vi "Trajectory Builder.vi"() -> ()   [LabVIEW 2020]
uses:
  Availible Command systems for auto.ctl
  <vilib>/event_ctls.llb/lveventtype.ctl
panel:
  out "Picture":picture
  in  "Initial Location":cluster{"x":dbl, "y":dbl, "th":dbl}[](array[cluster])=[{"x"=9.6, "y"=6.2, "th"=90.0}]
  out "appended path":path
  out "folder names":cluster{"name":string, "name":string}
  in  "Directory":bool
  in  "Tab Control":T1(tab)
  out "Duration (s)":dbl format="%#.4g"
  out "Distance (ft)":dbl format="%#.1g"
  out "WayPoints":cluster{"x":dbl, "y":dbl, "th":dbl}[](array[cluster]) {"th" format="%#_4g"}
  in  "Center Flip":bool
  in  "Snap to foot":bool
  in  "Angle Limiter":enum16{"90", "45", "15", "1"}(ring)=enum."15"
  in  "Snap robot to baseline":bool
  in  "Angular Accelerations":T2 {"Angular \nAccelerations" step=5.0}
  in  "Limits":T3={"Velocity (fps)"=6.0, "Accel (fps^2)"=15.0, "Jerk (fps^3)"=15.0} {"Jerk (fps^3)" min=0.0 step=1.0; "Accel (fps^2)" min=0.0; "Velocity (fps)" min=0.0}
  in  "Conditions":T4 {"vFinal (fps)" min=0.0; "vInitial (fps)" min=0.0}
  in  "Sample Period (s)":dbl=0.02
  in  "Unjank":bool
  in  "Turn \nAcceleration":bool=TRUE
  in  "Turn \nDeceleration":bool=TRUE
  out "Command Info":string
  in  "Reorder":bool
  in  "Commands":T5(array[cluster]) {"System" items=["Elevator", "Carriage Intake STOP", "Carriage Intake RUN"]}
  in  "Time (s)":dbl(slide) scale=-1.0..2.02 scale format="%#.1g"
  in  "Play":bool
  in  "Sub Dir 2":u16(ring)
  in  "Sub Dir 1":u16(ring) items=["Experimental", "Left", "Other", "Right"]
  out "fps":dbl[](graph)
  in  "Append":bool
  in  "Open":i32(listbox)
  in  "Filename":string
  in  "Save":bool
  in  "New":bool
  # "Directions:\nUse mouse to ...\n    move robot position (rectangle with arrow)\n    rotate robot (red arrow)\n    move waypoints (numbered circles)\nClick in open space to add a waypoint\nShift click to delete a waypoint\nHover over a waypoint and use arrow keys to nudge\n\nTime slider and Play button will run robot along path\nto test for collisions\n\nDirection and Destionation are folder selectors for files\n\nNew creates a new path at default location\n\nAppend creates a path"
  # "Nicotine"
  # "(20ms)"
  # "Interaction Options"
  # "Path Info"
  # "1"
  # "2"
  # "3"
  # "4"
  # "5"
  # "6"
  # "7"
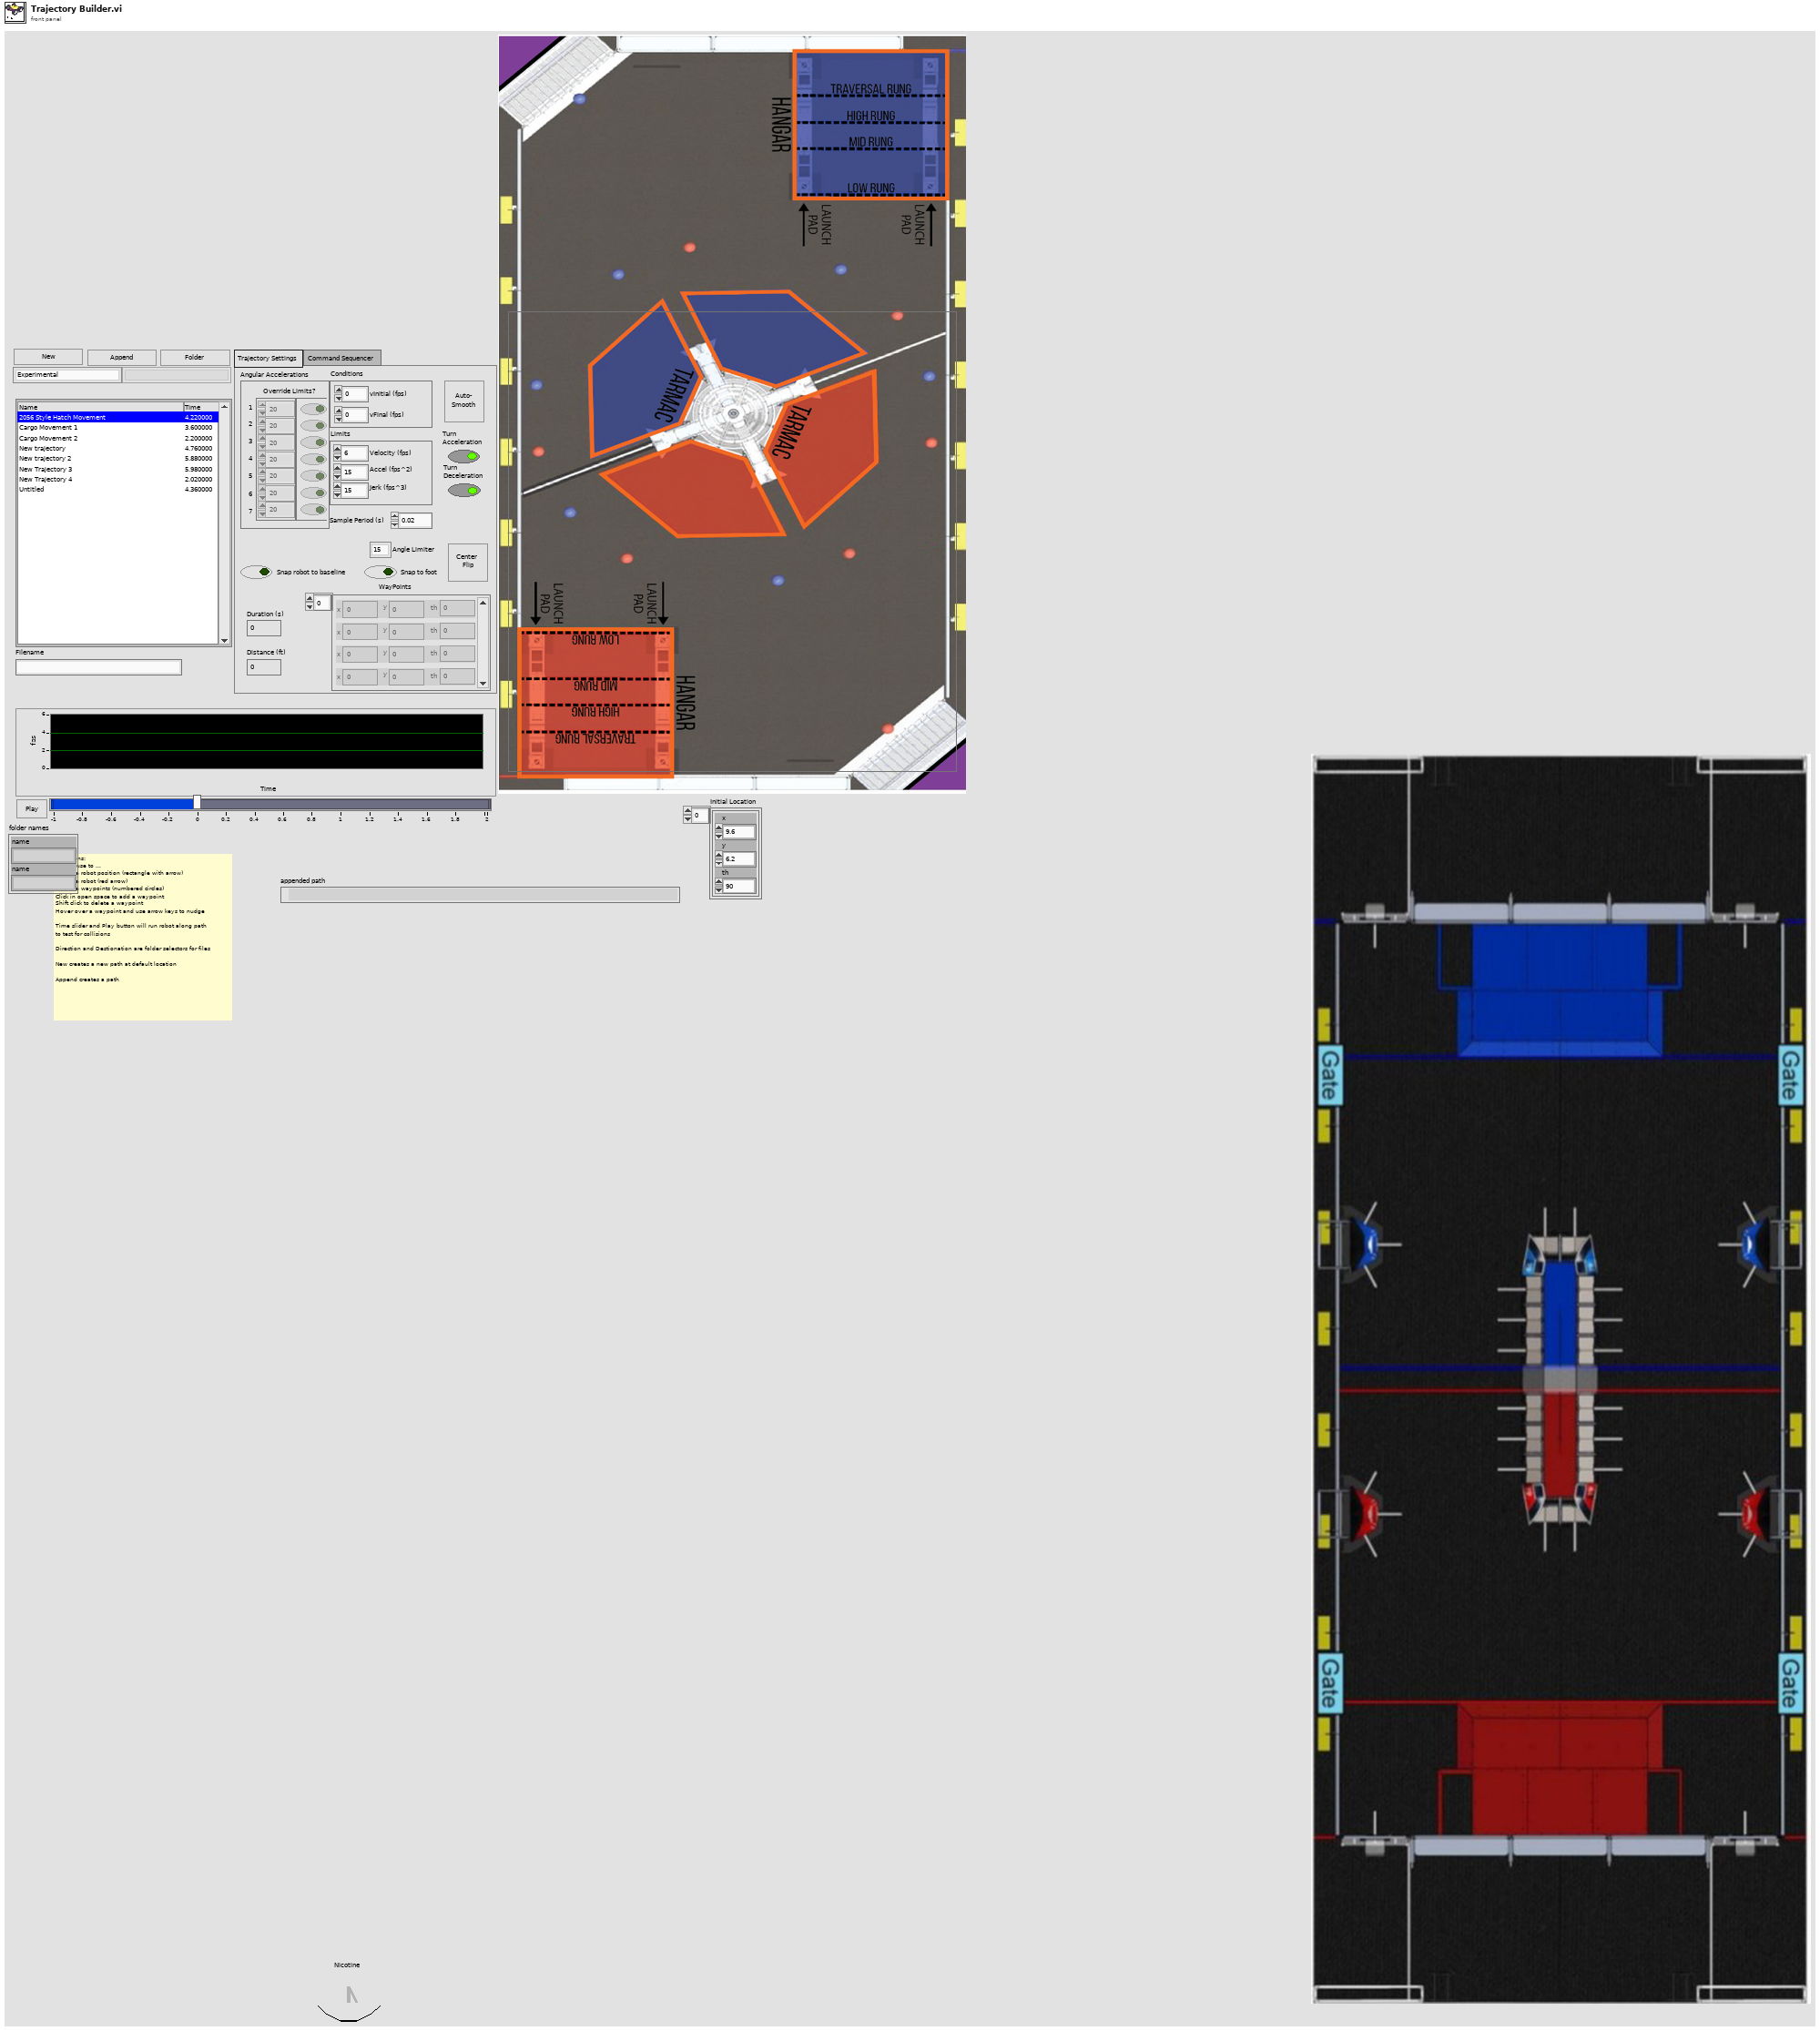
[diagram p1: front panel]
types:
  T1 = enum32{"Trajectory Settings", "Command Sequencer"}
  T2 = cluster{"Angular \nAccelerations":dbl[], "Override Limits?":bool[]}
  T3 = cluster{"Velocity (fps)":dbl, "Accel (fps^2)":dbl, "Jerk (fps^3)":dbl}
  T4 = cluster{"vInitial (fps)":dbl, "vFinal (fps)":dbl}
  T5 = cluster{"Time into Path":dbl, "System":u16, "Item Selected?":bool, "System Selection":u16}[]
  T6 = cluster{"Sample Period (s)":dbl, "Limits":cluster{"Velocity (fps)":dbl, "Acceleration (fps^2)":dbl, "Jerk (fps^3)":dbl}, "Conditions":cluster{"vInitial (fps)":dbl, "vFinal (fps)":dbl}, "output cluster":cluster{"Angular \nAccelerations":dbl[], "Override Limits?":bool[]}}
  T7 = cluster{"Segment Name":string, "Type":enum16{"Accel Straight", "Const Straight", "Blend", "Circle"}, "Traj Pos Points":cluster{"x":dbl, "y":dbl, "th":dbl}[], "Traj Vel Points":cluster{"V":dbl, "th":dbl}[], "Accel Index":i32, "Decel Index":i32}[]
  T8 = cluster{"Index":i32, "Pt Test Results":enum16{"Miss", "Rect Hit", "Arrow Hit"}}
  T9 = cluster{"Drag Object":cluster{"Index":i32, "x":dbl, "y":dbl}, "Hover Object":cluster{"Index":i32, "Pt Test Results":enum16{"Miss", "Rect Hit", "Arrow Hit"}}}
  T10 = cluster{"Trajectory Data":cluster{"Segment Name":string, "Type":enum16{"Accel Straight", "Const Straight", "Blend", "Circle"}, "Traj Pos Points":cluster{"x":dbl, "y":dbl, "th":dbl}[], "Traj Vel Points":cluster{"V":dbl, "th":dbl}[], "Accel Index":i32, "Decel Index":i32}[], "Points":cluster{"x":dbl, "y":dbl, "th":dbl}[], "Cluster":cluster{"Sample Period (s)":dbl, "Limits":cluster{"Velocity (fps)":dbl, "Acceleration (fps^2)":dbl, "Jerk (fps^3)":dbl}, "Conditions":cluster{"vInitial (fps)":dbl, "vFinal (fps)":dbl}, "output cluster":cluster{"Angular \nAccelerations":dbl[], "Override Limits?":bool[]}}}
  T11 = cluster{"Velocity":dbl, "Sample Time":dbl, "Accel":dbl}
  T12 = cluster{"Sample Period (s)":dbl, "Limits":cluster{"Velocity (fps)":dbl, "Acceleration (fps^2)":dbl, "Jerk (fps^3)":dbl}, "Conditions":cluster{"vInitial (fps)":dbl, "vFinal (fps)":dbl}}
  T13 = cluster{"Sample Period (s)":dbl, "Limits":cluster{"Velocity (fps)":dbl, "Acceleration (fps^2)":dbl, "Jerk (fps^3)":dbl}, "Conditions":cluster{"vInitial (fps)":dbl, "vFinal (fps)":dbl}, "Min Rads":dbl[]}
  T14 = typedef "Availible Command systems for auto.ctl" = u16
  T15 = cluster{"Time into Path":dbl, "System":T14, "Item Selected?":bool, "System Selection":T14}[]
  T16 = typedef "lveventtype.ctl" = enum32{"Null", "Timeout", "Annotation Menu Selection", "Annotation Menu Selection?", "App Instance Close", "App Instance Close?", "Autoscale Range Change", "Bookmark Info Change", "Cell Edit", "Cell Edit?", "Cursor Grab", "Cursor Grab?", "Cursor Menu Selection", "Cursor Menu Selection?", "Cursor Move", "Cursor Release", "Data Change", "Direction Change", "Display State Change", "Drag Ended", "Drag Enter", "Drag Leave", "Drag Over", "Drag Source Update", "Drag Starting", "Drag Starting?", "Drop", "Exec State Change", "Key Down", "Key Down?", "Key Repeat", "Key Repeat?", "Key Up", "Listbox Double Click", "Menu Activation?", "Menu Selection (App)", "Menu Selection? (App)", "Menu Selection (User)", "Mouse Down", "Mouse Down?", "Mouse Enter", "Mouse Leave", "Mouse Move", "Mouse Up", "Mouse Wheel", "NI Security User Change (App)", "Pane Size", "Panel Close", "Panel Close?", "Panel Resize", "Plot Attribute Change", "Scale Range Change", "Shortcut Menu Activation?", "Shortcut Menu Selection (App)", "Shortcut Menu Selection? (App)", "Shortcut Menu Selection (User)", "Tree Double Click", "Tree Drag", "Tree Drag?", "Tree Drop", "Tree Drop?", "Tree Item Close", "Tree Item Close?", "Tree Item Open", "Tree Item Open?", "User Event", "Value Change"}
  T17 = cluster{"Sample Period (s)":dbl, "Limits":cluster{"Velocity (fps)":dbl, "Accel (fps^2)":dbl, "Jerk (fps^3)":dbl}, "Conditions":cluster{"vInitial (fps)":dbl, "vFinal (fps)":dbl}, "Angular Accelerations":cluster{"Angular \nAccelerations":dbl[], "Override Limits?":bool[]}}
  T18 = typedef "LVPoint32TypeDef.ctl" = cluster{"Horizontal":i32, "Vertical":i32}
  T19 = cluster{"Shift":bool, "Ctrl":bool, "Alt":bool, "Cmd":bool, "Opt":bool}
  T20 = typedef "LVPositionTypeDef.ctl" = cluster{"Left":i32, "Top":i32}
  T21 = typedef "LVBoundsTypeDef.ctl" = cluster{"Width":u32, "Height":u32}
  T22 = cluster{"Velocity":dbl, "Accel":dbl, "Accel":dbl}
  T23 = cluster{"Velocity (fps)":dbl, "Acceleration (fps^2)":dbl, "Jerk (fps^3)":dbl}
  T24 = cluster{"Trajectory Data":cluster{"Segment Name":string, "Type":enum16{"Accel Straight", "Const Straight", "Blend", "Circle"}, "Traj Pos Points":cluster{"x":dbl, "y":dbl, "th":dbl}[], "Traj Vel Points":cluster{"V":dbl, "th":dbl}[], "Accel Index":i32, "Decel Index":i32}[], "Points":cluster{"x":dbl, "y":dbl, "th":dbl}[], cluster{"Sample Period (s)":dbl, "Limits":cluster{"Velocity (fps)":dbl, "Accel (fps^2)":dbl, "Jerk (fps^3)":dbl}, "Conditions":cluster{"vInitial (fps)":dbl, "vFinal (fps)":dbl}, "Angular Accelerations":cluster{"Angular \nAccelerations":dbl[], "Override Limits?":bool[]}}}
  T25 = cluster{"Snap robot to baseline":bool, "Snap to foot":bool, "Angle Limiter":enum16{"90", "45", "15", "1"}}
  T26 = cluster{i32, "Pt Test Results":enum16{"Miss", "Rect Hit", "Arrow Hit"}}
  T27 = cluster{"Drag Object":cluster{"Index":i32, "x":dbl, "y":dbl}, "Results":cluster{"Index":i32, "Pt Test Results":enum16{"Miss", "Rect Hit", "Arrow Hit"}}}
  T28 = cluster{"Trajectory Data":cluster{"Segment Name":string, "Type":enum16{"Accel Straight", "Const Straight", "Blend", "Circle"}, "Traj Pos Points":cluster{"x":dbl, "y":dbl, "th":dbl}[], "Traj Vel Points":cluster{"V":dbl, "th":dbl}[], "Accel Index":i32, "Decel Index":i32}[], "Updated Waypoints":cluster{"x":dbl, "y":dbl, "th":dbl}[], "Cluster":cluster{"Sample Period (s)":dbl, "Limits":cluster{"Velocity (fps)":dbl, "Accel (fps^2)":dbl, "Jerk (fps^3)":dbl}, "Conditions":cluster{"vInitial (fps)":dbl, "vFinal (fps)":dbl}, "Angular Accelerations":cluster{"Angular \nAccelerations":dbl[], "Override Limits?":bool[]}}}
  T29 = typedef "eventvkey.ctl" = enum16{"ASCII", "Enter", "Return", "Shift", "Ctrl", "Alt", "Cmd", "Opt", "Caps", "NumLock", "Clear", "Break", "Up", "Down", "Left", "Right", "Insert", "Delete", "Home", "End", "PageUp", "PageDown", "Escape", "Help", "Pause", "ScrollLock", "F1", "F2", "F3", "F4", "F5", "F6", "F7", "F8", "F9", "F10", "F11", "F12", "F13", "F14", "F15", "F16", "F17", "F18", "F19", "F20", "F21", "F22", "F23", "F24", "Play", "VolumeUp", "VolumeDown", "Mute", "Two Byte Char"}
  T30 = cluster{"Trajectory Data":cluster{"Segment Name":string, "Type":enum16{"Accel Straight", "Const Straight", "Blend", "Circle"}, "Traj Pos Points":cluster{"x":dbl, "y":dbl, "th":dbl}[], "Traj Vel Points":cluster{"V":dbl, "th":dbl}[], "Accel Index":i32, "Decel Index":i32}[], "Updated Waypoints":cluster{"x":dbl, "y":dbl, "th":dbl}[], cluster{"Sample Period (s)":dbl, "Limits":cluster{"Velocity (fps)":dbl, "Accel (fps^2)":dbl, "Jerk (fps^3)":dbl}, "Conditions":cluster{"vInitial (fps)":dbl, "vFinal (fps)":dbl}, "Angular Accelerations":cluster{"Angular \nAccelerations":dbl[], "Override Limits?":bool[]}}}
  T31 = cluster{"Horizontal":dbl, "Vertical":dbl, "th":dbl}
  T32 = cluster{"Name":string, "Color":u32, "Style":i32, "Point Style":i32, "Name Visible":bool, "Allow Drag":bool, "Annotation Mode":i32, "Plot":i32, "Index":i32, "Position":cluster{"X":dbl, "Y":dbl}, "X Scale":i32, "Y Scale":u32, "Show Arrow":bool, "Lock Name":bool, "Plot Area":i32, "Label Offset":cluster{"X":dbl, "Y":dbl}}[]
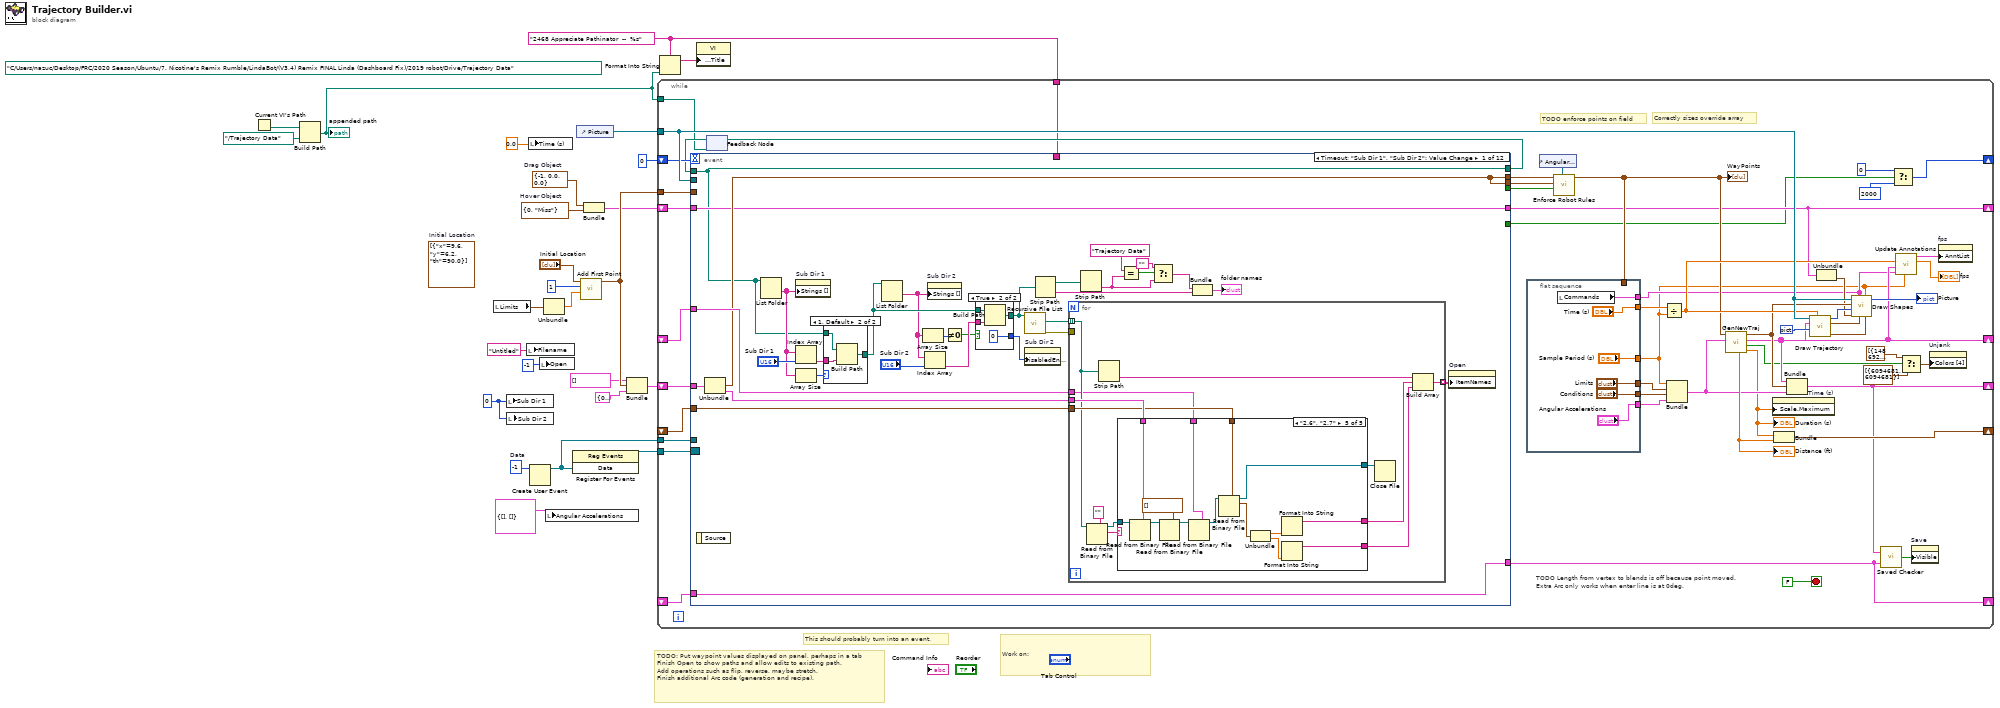
[diagram p0: block diagram]
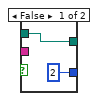
[diagram p3: hidden frame]
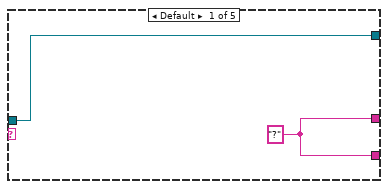
[diagram p4: hidden frame]
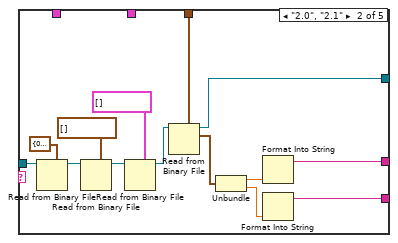
[diagram p5: hidden frame]
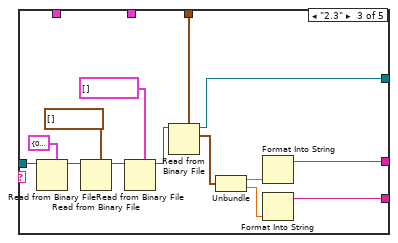
[diagram p6: hidden frame]
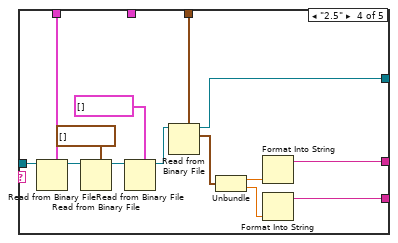
[diagram p7: hidden frame]
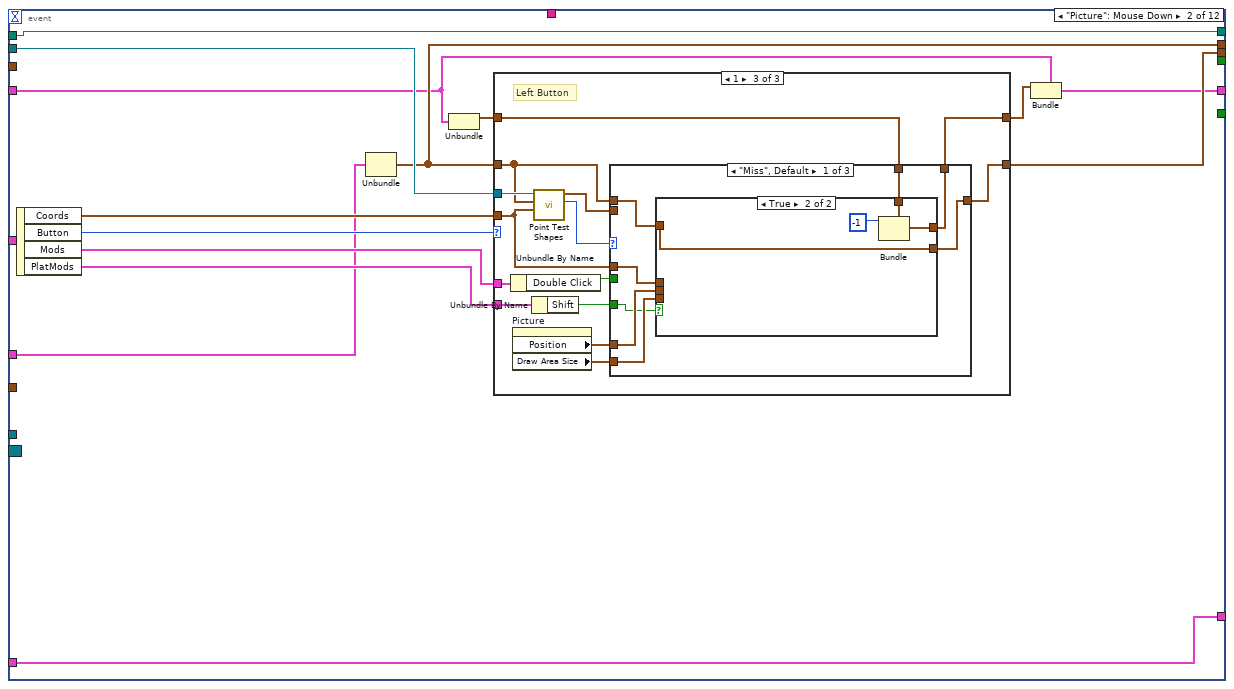
[diagram p8: hidden frame]
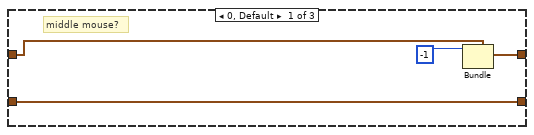
[diagram p9: hidden frame]
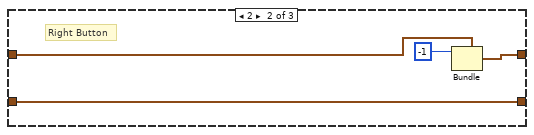
[diagram p10: hidden frame]
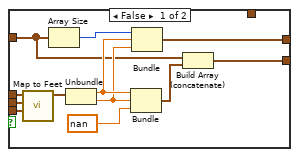
[diagram p11: hidden frame]
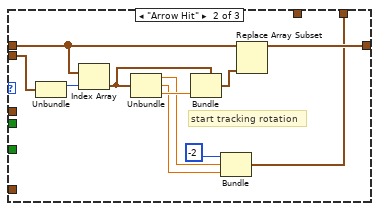
[diagram p12: hidden frame]
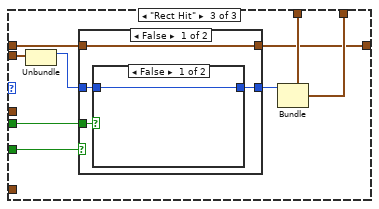
[diagram p13: hidden frame]
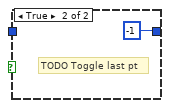
[diagram p14: hidden frame]
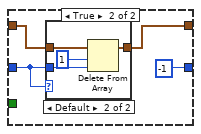
[diagram p15: hidden frame]
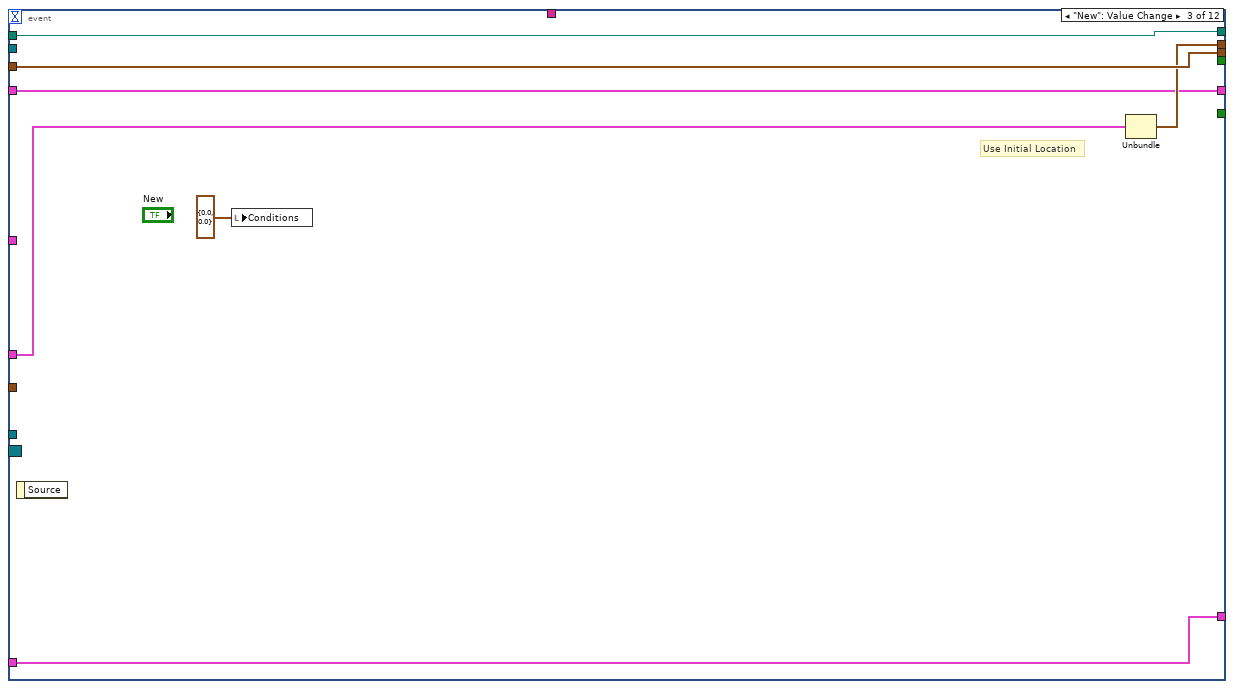
[diagram p17: hidden frame]
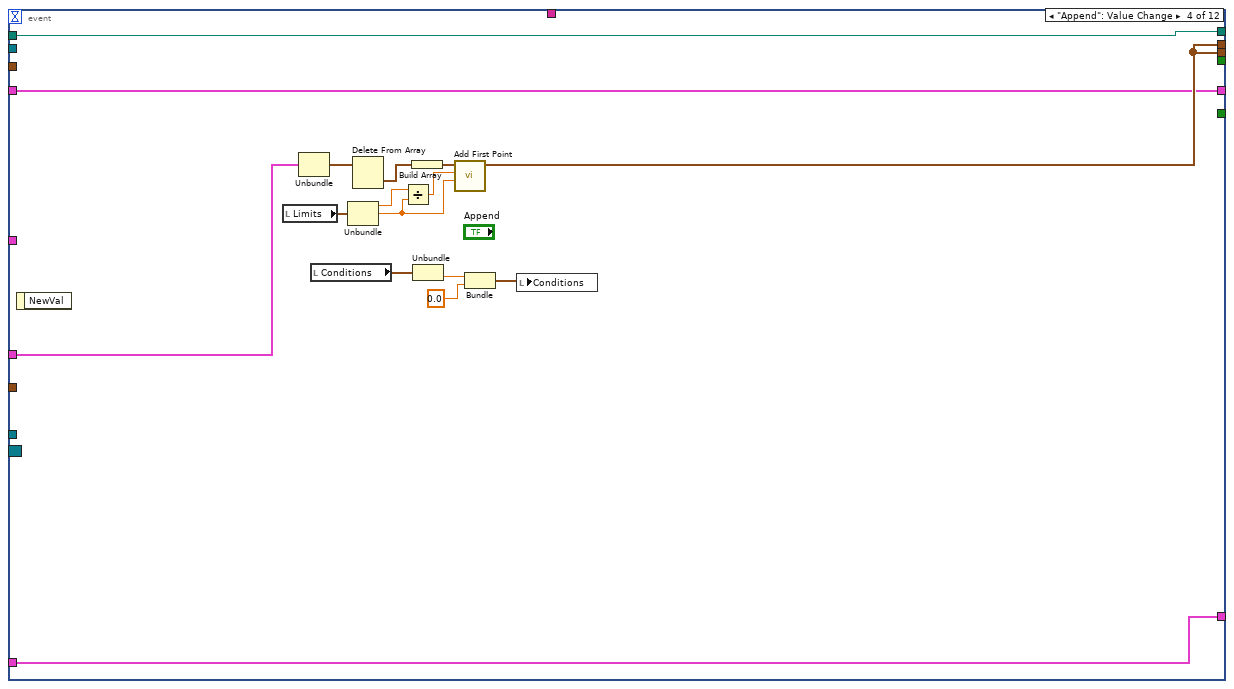
[diagram p18: hidden frame]
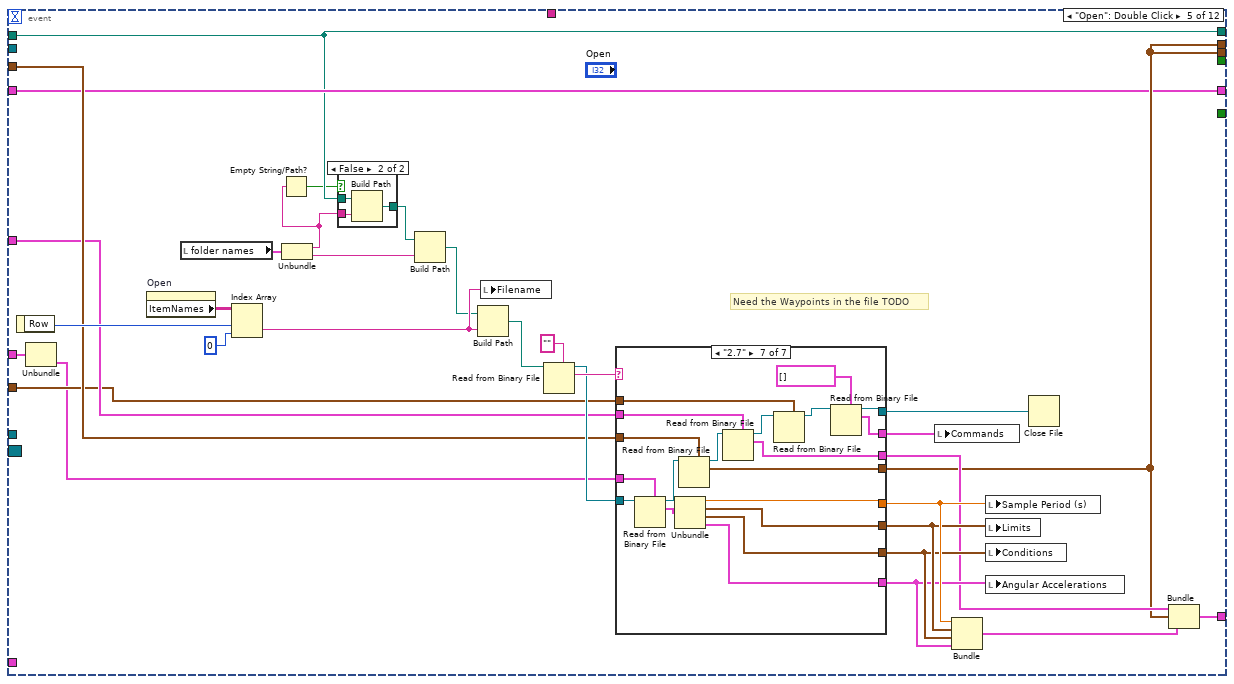
[diagram p19: hidden frame]
diagram:
  (unwired) cluster{"x":dbl, "y":dbl, "th":dbl}[] [{"x"=9.6, "y"=6.2, "th"=90.0}]  # Initial Location
  (unwired) path "C:/Users/nazuc/Desktop/FRC/2020 Season/Ubuntu/7. Nicotine's Remix Rumble/LindaBot/(V3.4) Remix FINAL Linda (Dashboard Fix)/2019 robot/Drive/Trajectory Data" ("Robot File")
  w4 = 0 ("th")
  w5 = "2468 Appreciate Pathinator  --  %s" ("format string")
  w15 = -1  # Data
  w9 = T8 {"Index"=0, "Pt Test Results"=enum."Miss"}  # Hover Object
  w8 = cluster{"Index":i32, "x":dbl, "y":dbl} {"Index"=-1, "x"=0.0, "y"=0.0}  # Drag Object
  # "This should probably turn into an event."
  # "Work on:"
  # "TODO: Put waypoint values displayed on panel, perhaps in a tab\nFinish Open to show paths and allow edits to existing path.\nAdd operations such as flip, reverse, maybe stretch.\nFinish additional Arc code (generation and recipe)."
  n1 = Current VI's Path() -> (path=w3:path)
  n2 = Build Path(base path=w3, name or relative path=path "../Trajectory Data") -> (appended path=w1:path)
  "appended path" <- w1
  n3 = local read "Limits"() -> (w21:T3)
  n4 = local write "Sub Dir 1"(w4) -> ()
  n5 = local write "Sub Dir 2"(w4) -> ()
  n6 = local write "Filename"("Untitled" ("Filename")) -> ()
  n7 = local write "Time (s)"(0.0 ("Time")) -> ()
  n8 = Create User Event(user event datatype=w15) -> (user event=w16:refnum<user-event>)  [unwired: 1 in, 1 out]
  n9 = local write "Open"(-1) -> ()
  n10 = Unbundle(w21) -> ("Accel (fps^2)"=w20:dbl)  [unwired: 2 out]
  n11 = local write "Angular Accelerations"(T2 {"Angular \nAccelerations"=[], "Override Limits?"=[]} ("Angular Accelerations")) -> ()
  n12 = register-events(w16) -> (reference out=w17:refnum<event-registration>)  [unwired: 2 in, 1 out]
  n13 = control-ref of="Picture"() -> (w26:refnum<vi>)
  n14 = call "Add First Point.vi"("Accel (f/s^2)"=w20, "Time (s)"=1 ("th"), "Initial Points"="Initial Location") -> ("Points"=w13:cluster{"x":dbl, "y":dbl, "th":dbl}[])  [unwired: 8 in]
  n15 = Bundle("Drag Object"=w8, "Hover Object"=w9) -> (w7:T9)  [unwired: 1 in]
  n16 = Bundle("Trajectory Data"=T7 [], "Points"=w13, "Cluster"=T6 {"Sample Period (s)"=0.02, "Limits"={"Velocity (fps)"=11.0, "Acceleration (fps^2)"=19.0, "Jerk (fps^3)"=150.0}, "Conditions"={"vInitial (fps)"=0.0, "vFinal (fps)"=0.0}, "output cluster"={"Angular \nAccelerations"=[], "Override Limits?"=[]}}) -> (w12:T10)  [unwired: 1 in]
  n17 = while {
    tunnel: w13 -> [w78]
    tunnel: w26 -> [w77]
    shift-right: [w42] -> _
    shift-left: _ -> [w71]
    shift-right: [w35] -> _
    shift-left: 0 -> [w70]
    shift-right: [w69] -> _
    shift-left: _ -> [w68]
    tunnel: w1 -> [w48]
    tunnel: w17 -> [w61]
    tunnel: w16 -> [w60]
    shift-right: [w58] -> _
    shift-left: _ -> [w59]
    shift-right: [w47] -> _
    shift-left: w12 -> [w46]
    shift-right: [w40] -> _
    shift-left: w7 -> [w41]
    tunnel: w5 -> [w38]
    stop <- FALSE stop-if-true
    # "Correctly sizes override array"
    # "TODO Length from vertex to blends is off because point moved.\nExtra Arc only works when enter line is at 0deg."
    # "TODO enforce points on field"
    n18 = feedback #1(w48) -> (w49:path)
    n19 = event shown="[0] Timeout;  \"Sub Dir 1\", \"Sub Dir 2\": Value Change" {
      selector: w61 -> [_ _ _ _ _ _ _ _ _ _ _ _]
      dyn-events: _ -> [_ _ _ _ _ _ _ _ _ _ _ _]
      timeout: w70 -> [_ _ _ _ _ _ _ _ _ _ _ _]
      tunnel: [w97 w207 w298 w313 w325 w473 w510 w543 w577 w598 w605 w634] -> w67
      tunnel: w78 -> [_ _ w298 _ w339 _ _ _ _ _ _ _]
      tunnel: w77 -> [_ w206 _ _ _ w474 _ _ w564 _ _ _]
      tunnel: w71 -> [w101 _ _ _ w338 _ w517 _ _ _ _ _]
      tunnel: w49 -> [w95 w204 w296 w302 w317 w467 w503 w538 w578 w603 w621 w627]
      tunnel: [w97 w201 w293 w313 w325 w464 w510 w534 w562 w598 w605 w634] -> w66
      tunnel: w68 -> [w114 _ _ _ w336 _ w522 _ _ _ _ _]
      tunnel: [_ _ _ _ _ _ _ TRUE ("Flip Over Center") _ _ _ _] -> w65
      tunnel: [w95 w204 w296 w302 w317 w467 w503 w538 w578 w603 w621 w625] -> w50
      tunnel: w60 -> [_ _ _ _ _ _ _ _ _ w602 w620 _]
      tunnel: [w107 w203 w295 w303 w328 w466 w518 w537 w565 w601 w617 w636] -> w58
      tunnel: w59 -> [w107 w203 w295 w303 _ w466 _ w537 w565 w601 w617 w636]
      tunnel: w46 -> [w99 w202 w294 w301 w324 w465 w513 w535 w563 w599 w606 w635]
      tunnel: w41 -> [w96 w198 w292 w299 w322 w460 w511 w533 w560 w597 w604 w637]
      tunnel: [w96 w200 w292 w299 w322 w461 w511 w533 w560 w597 w604 w637] -> w40
      tunnel: w38 -> [_ _ _ _ _ _ _ _ _ _ _ w631]
      tunnel: [_ _ _ _ _ _ TRUE _ _ _ _ TRUE] -> w34
      event Timeout; "Sub Dir 1", "Sub Dir 2": Value Change {
        n20 = event-data() -> ()  [unwired: 1 in, 1 out]
        n21 = Unbundle(w99) -> ("Updated Waypoints"=w97:cluster{"x":dbl, "y":dbl, "th":dbl}[], "Cluster"=w98:T17)  [unwired: 1 out]
        n22 = List Folder(path=w95) -> (folder names=w103:string[])  [unwired: 3 in, 3 out]
        n23 = Index Array(array=w103, index="Sub Dir 1") -> (element=w104:string)
        n24 = Array Size(array=w103) -> (size(s)=w100:i32)
        n25 = property on="Sub Dir 1" class="Ring (strict)"("Strings []"=w103) -> ()  [unwired: 2 in, 2 out]
        n26 = case shown="1, Default" w100 {
          tunnel: w95 -> [w117 w120]
          tunnel: [w117 w119] -> w105
          tunnel: w104 -> [_ w118]
          frame 0 {
          }
          frame 1, Default {
            n27 = Build Path(base path=w120, name or relative path=w118) -> (appended path=w119:path)
          }
        }
        n28 = List Folder(path=w105) -> (folder names=w102:string[])  [unwired: 3 in, 3 out]
        n29 = Array Size(array=w102) -> (size(s)=w106:i32)
        n30 = Index Array(array=w102, index="Sub Dir 2") -> (element=w110:string)
        n31 = property on="Sub Dir 2" class="Ring (strict)"("Strings []"=w102) -> ()  [unwired: 2 in, 2 out]
        n32 = Not Equal To 0?(x=w106) -> (x != 0?=w109:bool)
        n33 = case shown="True" w109 {
          tunnel: w105 -> [w122 w126]
          tunnel: [w122 w125] -> w94
          tunnel: w110 -> [_ w124]
          tunnel: [2 0] -> w108
          frame False {
          }
          frame True {
            n34 = Build Path(base path=w126, name or relative path=w124) -> (appended path=w125:path)
          }
        }
        n35 = call <vilib>:"Recursive File List.vi"("Folder Path"=w94) -> ("error out"=w113:errorcluster, "All Files in Dir"=w116:path[])  [unwired: 6 in, 3 out]
        n36 = property on="Sub Dir 2" class="Ring (strict)"("DisabledEnum"=w108) -> ()  [unwired: 2 in, 2 out]
        n37 = Strip Path(path=w94) -> (stripped path=w93:path, name=w91:string)
        n38 = for {
          tunnel: w116 -> [w128] mode=indexing
          tunnel: [w138] -> w115 mode=indexing
          tunnel: w98 -> [w133]
          tunnel: w114 -> [w132]
          tunnel: w113 -> [_]
          tunnel: w101 -> [w127]
          n39 = Read from Binary File(5:"", 11:w128) -> (2:w136:string, 3:w135:refnum<file>)  [unwired: 4 in, 2 out]
          n40 = Strip Path(path=w128) -> (name=w129:string)  [unwired: 1 out]
          n41 = case shown="\"2.6\", \"2.7\"" w136 {
            tunnel: [w140 w154 w168 w182 w196] -> w131
            tunnel: [w140 w153 w167 w181 w195] -> w130
            tunnel: w135 -> [w139 w152 w166 w180 w194]
            tunnel: [w139 w148 w162 w176 w190] -> w134
            tunnel: w133 -> [_ _ _ w169 w184]
            tunnel: w132 -> [_ w147 w161 w175 w189]
            tunnel: w127 -> [_ _ _ _ w183]
            frame Default {
              w140 = "?"
            }
            frame "2.0", "2.1" {
              n42 = Read from Binary File(5:T11 {"Velocity"=0.0, "Sample Time"=0.0, "Accel"=0.0}, 11:w152) -> (3:w151:refnum<file>)  [unwired: 4 in, 3 out]
              n43 = Read from Binary File(5:cluster{"x":dbl, "y":dbl, "th":dbl}[] [] ("Points"), 11:w151) -> (3:w150:refnum<file>)  [unwired: 4 in, 3 out]
              n44 = Read from Binary File(5:T7 [] ("Trajectory Data"), 11:w150) -> (3:w149:refnum<file>)  [unwired: 4 in, 3 out]
              n45 = Read from Binary File(5:w147, 11:w149) -> (2:w142:cluster{"Time (s)":dbl, "Distance (ft)":dbl}, 3:w148:refnum<file>)  [unwired: 4 in, 2 out]
              n46 = Unbundle(w142) -> ("Time (s)"=w146:dbl, "Distance (ft)"=w145:dbl)
              n47 = Format Into String(w146) -> (resulting string=w154:string)  [unwired: 3 in, 1 out]
              n48 = Format Into String(w145) -> (resulting string=w153:string)  [unwired: 3 in, 1 out]
            }
            frame "2.3" {
              n49 = Read from Binary File(5:T12 {"Sample Period (s)"=0.0, "Limits"={"Velocity (fps)"=0.0, "Acceleration (fps^2)"=0.0, "Jerk (fps^3)"=0.0}, "Conditions"={"vInitial (fps)"=0.0, "vFinal (fps)"=0.0}}, 11:w166) -> (3:w165:refnum<file>)  [unwired: 4 in, 3 out]
              n50 = Read from Binary File(5:cluster{"x":dbl, "y":dbl, "th":dbl}[] [] ("Points"), 11:w165) -> (3:w164:refnum<file>)  [unwired: 4 in, 3 out]
              n51 = Read from Binary File(5:T7 [] ("Trajectory Data"), 11:w164) -> (3:w163:refnum<file>)  [unwired: 4 in, 3 out]
              n52 = Read from Binary File(5:w161, 11:w163) -> (2:w156:cluster{"Time (s)":dbl, "Distance (ft)":dbl}, 3:w162:refnum<file>)  [unwired: 4 in, 2 out]
              n53 = Unbundle(w156) -> ("Time (s)"=w160:dbl, "Distance (ft)"=w159:dbl)
              n54 = Format Into String(w160) -> (resulting string=w168:string)  [unwired: 3 in, 1 out]
              n55 = Format Into String(w159) -> (resulting string=w167:string)  [unwired: 3 in, 1 out]
            }
            frame "2.5" {
              n56 = Read from Binary File(5:w169, 11:w180) -> (3:w179:refnum<file>)  [unwired: 4 in, 3 out]
              n57 = Read from Binary File(5:cluster{"x":dbl, "y":dbl, "th":dbl}[] [] ("Points"), 11:w179) -> (3:w178:refnum<file>)  [unwired: 4 in, 3 out]
              n58 = Read from Binary File(5:T7 [] ("Trajectory Data"), 11:w178) -> (3:w177:refnum<file>)  [unwired: 4 in, 3 out]
              n59 = Read from Binary File(5:w175, 11:w177) -> (2:w170:cluster{"Time (s)":dbl, "Distance (ft)":dbl}, 3:w176:refnum<file>)  [unwired: 4 in, 2 out]
              n60 = Unbundle(w170) -> ("Time (s)"=w174:dbl, "Distance (ft)"=w173:dbl)
              n61 = Format Into String(w174) -> (resulting string=w182:string)  [unwired: 3 in, 1 out]
              n62 = Format Into String(w173) -> (resulting string=w181:string)  [unwired: 3 in, 1 out]
            }
            frame "2.6", "2.7" {
              n63 = Read from Binary File(5:w184, 11:w194) -> (3:w193:refnum<file>)  [unwired: 4 in, 3 out]
              n64 = Read from Binary File(5:cluster{"x":dbl, "y":dbl, "th":dbl}[] [] ("Points"), 11:w193) -> (3:w192:refnum<file>)  [unwired: 4 in, 3 out]
              n65 = Read from Binary File(5:w183, 11:w192) -> (3:w191:refnum<file>)  [unwired: 4 in, 3 out]
              n66 = Read from Binary File(5:w189, 11:w191) -> (2:w185:cluster{"Time (s)":dbl, "Distance (ft)":dbl}, 3:w190:refnum<file>)  [unwired: 4 in, 2 out]
              n67 = Unbundle(w185) -> ("Time (s)"=w188:dbl, "Distance (ft)"=w187:dbl)
              n68 = Format Into String(w188) -> (resulting string=w196:string)  [unwired: 3 in, 1 out]
              n69 = Format Into String(w187) -> (resulting string=w195:string)  [unwired: 3 in, 1 out]
            }
          }
          n70 = Close File(refnum=w134) -> ()  [unwired: 1 in, 2 out]
          n71 = Build Array(w129, w131, w130) -> (w138:string[])
        }
        n72 = Strip Path(path=w93) -> (name=w87:string)  [unwired: 1 out]
        n73 = Equal?(x="Trajectory Data", y=w87) -> (x = y?=w90:bool)
        n74 = Select(t="", s=w90, f=w87) -> (s? t:f=w86:string)
        n75 = Bundle("name"=w86, "name"=w91) -> (→"folder names":cluster{"name":string, "name":string})  [unwired: 1 in]
        n76 = property on="Open" class="MCListbox (strict)"("ItemNames"=w115) -> ()  [unwired: 2 in, 2 out]
      }
      event "Picture": Mouse Down {
        n77 = event-data() -> ("Coords"=w208:T18, "Button"=w210:u16, "Mods"=w209:cluster{"Double Click":bool, "Menu Key":bool}, "PlatMods"=w205:T19)  [unwired: 1 in]
        n78 = Unbundle(w202) -> ("Updated Waypoints"=w201:cluster{"x":dbl, "y":dbl, "th":dbl}[])  [unwired: 2 out]
        n79 = Unbundle(w198) -> ("Drag Object"=w197:cluster{"Index":i32, "x":dbl, "y":dbl})  [unwired: 1 out]
        n80 = case shown="1" w210 {
          tunnel: w209 -> [_ _ w222]
          tunnel: w208 -> [_ _ w227]
          tunnel: w201 -> [w214 w218 w228]
          tunnel: [w214 w218 w232] -> w207
          tunnel: w206 -> [_ _ w229]
          tunnel: w197 -> [w212 w215 w223]
          tunnel: [w211 w217 w224] -> w199
          tunnel: w205 -> [_ _ w220]
          frame 0, Default {
            # "middle mouse?"
            n81 = Bundle(cluster=w212, "Index"=-1) -> (w211:cluster{"Index":i32, "x":dbl, "y":dbl})  [unwired: 2 in]
          }
          frame 2 {
            # "Right Button"
            n82 = Bundle(cluster=w215, "Index"=-1) -> (w217:cluster{"Index":i32, "x":dbl, "y":dbl})  [unwired: 2 in]
          }
          frame 1 {
            # "Left Button"
            n83 = Unbundle By Name(w222) -> ("Double Click"=w221:bool)
            n84 = property on="Picture" class="Pict"() -> ("Position"=w231:T20, "Draw Area Size"=w230:T21)  [unwired: 2 in, 2 out]
            n85 = Unbundle By Name(w220) -> ("Shift"=w219:bool)
            n86 = call "Point Test Shapes.vi"("Coords"=w227, "Points"=w228, "Picture in"=w229) -> ("Pt Test Results"=w226:enum16{"Miss", "Rect Hit", "Arrow Hit"}, "Results"=w225:T8)  [unwired: 7 in]
            n87 = case shown="\"Miss\", Default" w226 {
              tunnel: w221 -> [_ _ w275]
              tunnel: w228 -> [w236 w264 w269]
              tunnel: w225 -> [_ w262 w276]
              tunnel: [w239 w265 w268] -> w232
              tunnel: w227 -> [w240 _ _]
              tunnel: w231 -> [w238 _ _]
              tunnel: w230 -> [w237 _ _]
              tunnel: [w234 w257 w272] -> w224
              tunnel: w223 -> [w233 _ w273]
              tunnel: w219 -> [w235 _ w270]
              frame "Miss", Default {
                n88 = case shown="True" w235 {
                  tunnel: w240 -> [w252 _]
                  tunnel: [w249 w256] -> w239
                  tunnel: w238 -> [w248 _]
                  tunnel: w237 -> [w247 _]
                  tunnel: w236 -> [w243 w256]
                  tunnel: [w242 w255] -> w234
                  tunnel: w233 -> [_ w253]
                  frame False {
                    n89 = call "Map to Feet.vi"("Draw Area Size"=w247, "Position"=w248, "Coords (px)"=w252) -> ("Point (ft)"=w246:cluster{dbl, dbl})  [unwired: 8 in]
                    n90 = Array Size(array=w243) -> (size(s)=w241:i32)
                    n91 = Unbundle(w246) -> (w245:dbl, w244:dbl)
                    n92 = Bundle(w245, w244, nan) -> (w250:cluster{dbl, dbl, dbl})  [unwired: 1 in]
                    n93 = Bundle(w241, w245, w244) -> (w242:cluster{i32, dbl, dbl})  [unwired: 1 in]
                    n94 = Build Array (concatenate)(w243, w250) -> (w249:cluster{"x":dbl, "y":dbl, "th":dbl}[])
                  }
                  frame True {
                    n95 = Bundle(cluster=w253, "Index"=-1) -> (w255:cluster{"Index":i32, "x":dbl, "y":dbl})  [unwired: 2 in]
                  }
                }
              }
              frame "Arrow Hit" {
                # "start tracking rotation"
                n96 = Unbundle(w262) -> ("Index"=w261:i32)  [unwired: 1 out]
                n97 = Index Array(array=w264, index=w261) -> (element=w263:cluster{"x":dbl, "y":dbl, "th":dbl})
                n98 = Unbundle(w263) -> ("x"=w260:dbl, "y"=w259:dbl, "th"=w267:dbl)
                n99 = Bundle(cluster=w263, "th"=w267) -> (w266:cluster{"x":dbl, "y":dbl, "th":dbl})  [unwired: 2 in]
                n100 = Bundle(-2, "x"=w260, "y"=w259) -> (w257:cluster{i32, "x":dbl, "y":dbl})  [unwired: 1 in]
                n101 = Replace Array Subset(array=w264, new element=w266) -> (w265:cluster{"x":dbl, "y":dbl, "th":dbl}[])  [unwired: 1 in]
              }
              frame "Rect Hit" {
                n102 = Unbundle(w276) -> ("Index"=w274:i32)  [unwired: 1 out]
                n103 = case shown="False" w270 {
                  tunnel: w275 -> [w280 _]
                  tunnel: w274 -> [w279 w283]
                  tunnel: [w278 -1 ("length")] -> w271
                  tunnel: w269 -> [w277 w286]
                  tunnel: [w277 w285] -> w268
                  frame False {
                    n104 = case shown="False" w280 {
                      tunnel: w279 -> [w281 _]
                      tunnel: [w281 -1] -> w278
                      frame False {
                      }
                      frame True {
                        # "TODO Toggle last pt"
                      }
                    }
                  }
                  frame True {
                    n105 = case shown="Default" w283 {
                      tunnel: w286 -> [w287 w291]
                      tunnel: w283 -> [_ w290]
                      tunnel: [w287 w288] -> w285
                      frame 0 {
                      }
                      frame Default {
                        n106 = Delete From Array(array=w291, length=1, index=w290) -> (array with subset deleted=w288:cluster{"x":dbl, "y":dbl, "th":dbl}[])  [unwired: 1 out]
                      }
                    }
                  }
                }
                n107 = Bundle(cluster=w273, "Index"=w271) -> (w272:cluster{"Index":i32, "x":dbl, "y":dbl})  [unwired: 2 in]
              }
            }
          }
        }
        n108 = Bundle(cluster=w198, "Drag Object"=w199) -> (w200:T9)  [unwired: 1 in]
      }
      event "New": Value Change {
        # "Use Initial Location"
        n109 = event-data() -> ()  [unwired: 1 in, 1 out]
        n110 = local write "Conditions"(T4 {"vInitial (fps)"=0.0, "vFinal (fps)"=0.0} ("Conditions")) -> ()
        n111 = Unbundle(w294) -> ("Updated Waypoints"=w293:cluster{"x":dbl, "y":dbl, "th":dbl}[])  [unwired: 2 out]
      }
      event "Append": Value Change {
        n112 = event-data() -> ()  [unwired: 1 in, 1 out]
        n113 = local read "Limits"() -> (w306:T3)
        n114 = Unbundle(w301) -> ("Updated Waypoints"=w300:cluster{"x":dbl, "y":dbl, "th":dbl}[])  [unwired: 2 out]
        n115 = local read "Conditions"() -> (w310:T4)
        n116 = Unbundle(w306) -> ("Velocity (fps)"=w305:dbl, "Accel (fps^2)"=w304:dbl)  [unwired: 1 out]
        n117 = Delete From Array(array=w300) -> (deleted portion=w312:cluster{"x":dbl, "y":dbl, "th":dbl})  [unwired: 2 in, 1 out]
        n118 = Divide(x=w305, y=w304) -> (x/y=w314:dbl)
        n119 = Build Array(w312) -> (w311:cluster{"x":dbl, "y":dbl, "th":dbl}[])
        n120 = Unbundle(w310) -> ("vFinal (fps)"=w309:dbl)  [unwired: 1 out]
        n121 = call "Add First Point.vi"("Accel (f/s^2)"=w304, "Time (s)"=w314, "Initial Points"=w311) -> ("Points"=w313:cluster{"x":dbl, "y":dbl, "th":dbl}[])  [unwired: 8 in]
        n122 = Bundle("vFinal (fps)"=w309, 0.0) -> (w308:cluster{"vFinal (fps)":dbl, dbl})  [unwired: 1 in]
        n123 = local write "Conditions"(w308) -> ()
      }
      event "Open": Double Click {
        # "Need the Waypoints in the file TODO"
        n124 = event-data() -> ("Row"=w344:i32)  [unwired: 1 in]
        n125 = Unbundle(w324) -> ("Cluster"=w323:T17)  [unwired: 2 out]
        n126 = property on="Open" class="MCListbox (strict)"() -> ("ItemNames"=w345:string[][])  [unwired: 2 in, 2 out]
        n127 = local read "folder names"() -> (w321:cluster{"name":string, "name":string})
        n128 = Index Array(array=w345, index (row)=w344, index (col)=0 ("disabled index (col)")) -> (element=w334:string)
        n129 = Unbundle(w321) -> ("name"=w316:string, "name"=w319:string)
        n130 = Empty String/Path?(string/path=w316) -> (empty?=w315:bool)
        n131 = case shown="False" w315 {
          tunnel: w316 -> [_ w349]
          tunnel: [w346 w348] -> w320
          tunnel: w317 -> [w346 w347]
          frame True {
          }
          frame False {
            n132 = Build Path(base path=w347, name or relative path=w349) -> (appended path=w348:path)
          }
        }
        n133 = Build Path(base path=w320, name or relative path=w319) -> (appended path=w318:path)
        n134 = Build Path(base path=w318, name or relative path=w334) -> (appended path=w335:path)
        n135 = local write "Filename"(w334) -> ()
        n136 = Read from Binary File(5:"", 11:w335) -> (2:w341:string, 3:w340:refnum<file>)  [unwired: 4 in, 2 out]
        n137 = case shown="\"2.7\"" w341 {
          tunnel: w340 -> [w352 w369 w385 w401 w421 w438 w457]
          tunnel: w323 -> [_ _ _ _ _ w427 w447]
          tunnel: w339 -> [_ w367 w383 w399 w419 w436 w455]
          tunnel: [_ w366 w382 w398 w418 w435 w454] -> w325
          tunnel: w338 -> [_ w365 w381 w397 w417 w434 w453]
          tunnel: w336 -> [_ w363 w379 w395 w415 w432 w451]
          tunnel: [w352 w361 w377 w393 w413 w430 w442] -> w337
          tunnel: [_ w359 w376 w392 w412 w429 w449] -> w333
          tunnel: [_ w358 w375 w391 w411 w428 w448] -> w332
          tunnel: [_ _ w374 w390 w410 w426 w446] -> w331
          tunnel: [T2 {"Angular \nAccelerations"=[], "Override Limits?"=[]} ("Angular Accelerations") T2 {"Angular \nAccelerations"=[], "Override Limits?"=[]} ("Angular Accelerations") T2 {"Angular \nAccelerations"=[], "Override Limits?"=[]} ("Angular Accelerations") T2 {"Angular \nAccelerations"=[], "Override Limits?"=[]} ("Angular Accelerations") w404 w425 w445] -> w330
          tunnel: [T7 [] ("Trajectory Data") w353 w371 w387 w403 w424 w444] -> w327
          tunnel: [_ _ _ _ _ _ w441] -> w326
          frame "False", Default {
          }
          frame "2.0", "2.1" {
            n138 = Read from Binary File(5:T11 {"Velocity"=0.0, "Sample Time"=0.0, "Accel"=0.0}, 11:w369) -> (2:w370:T11, 3:w368:refnum<file>)  [unwired: 4 in, 2 out]
            n139 = Read from Binary File(5:w367, 11:w368) -> (2:w366:cluster{"x":dbl, "y":dbl, "th":dbl}[], 3:w364:refnum<file>)  [unwired: 4 in, 2 out]
            n140 = Unbundle(w370) -> ("Velocity"=w357:dbl, "Sample Time"=w359:dbl, "Accel"=w356:dbl)
            n141 = Read from Binary File(5:w365, 11:w364) -> (2:w353:T7, 3:w362:refnum<file>)  [unwired: 4 in, 2 out]
            n142 = Read from Binary File(5:w363, 11:w362) -> (3:w361:refnum<file>)  [unwired: 4 in, 3 out]
            n143 = Bundle("Velocity"=w357, "Accel"=w356, "Accel"=1000.0) -> (w358:T22)  [unwired: 1 in]
          }
          frame "2.3" {
            n144 = Read from Binary File(5:T12 {"Sample Period (s)"=0.0, "Limits"={"Velocity (fps)"=0.0, "Acceleration (fps^2)"=0.0, "Jerk (fps^3)"=0.0}, "Conditions"={"vInitial (fps)"=0.0, "vFinal (fps)"=0.0}}, 11:w385) -> (2:w386:T12, 3:w384:refnum<file>)  [unwired: 4 in, 2 out]
            n145 = Unbundle(w386) -> ("Sample Period (s)"=w376:dbl, "Limits"=w375:T23, "Conditions"=w374:T4)
            n146 = Read from Binary File(5:w383, 11:w384) -> (2:w382:cluster{"x":dbl, "y":dbl, "th":dbl}[], 3:w380:refnum<file>)  [unwired: 4 in, 2 out]
            n147 = Read from Binary File(5:w381, 11:w380) -> (2:w371:T7, 3:w378:refnum<file>)  [unwired: 4 in, 2 out]
            n148 = Read from Binary File(5:w379, 11:w378) -> (3:w377:refnum<file>)  [unwired: 4 in, 3 out]
          }
          frame "2.4" {
            n149 = Read from Binary File(5:T12 {"Sample Period (s)"=0.0, "Limits"={"Velocity (fps)"=0.0, "Acceleration (fps^2)"=0.0, "Jerk (fps^3)"=0.0}, "Conditions"={"vInitial (fps)"=0.0, "vFinal (fps)"=0.0}}, 11:w401) -> (2:w402:T12, 3:w400:refnum<file>)  [unwired: 4 in, 2 out]
            n150 = Unbundle(w402) -> ("Sample Period (s)"=w392:dbl, "Limits"=w391:T23, "Conditions"=w390:T4)
            n151 = Read from Binary File(5:w399, 11:w400) -> (2:w398:cluster{"x":dbl, "y":dbl, "th":dbl}[], 3:w396:refnum<file>)  [unwired: 4 in, 2 out]
            n152 = Read from Binary File(5:w397, 11:w396) -> (2:w387:T7, 3:w394:refnum<file>)  [unwired: 4 in, 2 out]
            n153 = Read from Binary File(5:w395, 11:w394) -> (3:w393:refnum<file>)  [unwired: 4 in, 3 out]
          }
          frame "2.5" {
            n154 = Read from Binary File(5:T13 {"Sample Period (s)"=0.0, "Limits"={"Velocity (fps)"=0.0, "Acceleration (fps^2)"=0.0, "Jerk (fps^3)"=0.0}, "Conditions"={"vInitial (fps)"=0.0, "vFinal (fps)"=0.0}, "Min Rads"=[20.0, 20.0, 20.0, 20.0, 20.0]}, 11:w421) -> (2:w422:T13, 3:w420:refnum<file>)  [unwired: 4 in, 2 out]
            n155 = Unbundle(w422) -> ("Sample Period (s)"=w412:dbl, "Limits"=w411:T23, "Conditions"=w410:T4, "Min Rads"=w406:dbl[])
            n156 = Array Size(array=w406) -> (size(s)=w407:i32)
            n157 = for {
              N: w407 -> [_]
              tunnel: [TRUE] -> w405 mode=indexing
            }
            n158 = Read from Binary File(5:w419, 11:w420) -> (2:w418:cluster{"x":dbl, "y":dbl, "th":dbl}[], 3:w416:refnum<file>)  [unwired: 4 in, 2 out]
            n159 = Read from Binary File(5:w417, 11:w416) -> (2:w403:T7, 3:w414:refnum<file>)  [unwired: 4 in, 2 out]
            n160 = Bundle(cluster=T2 {"Angular \nAccelerations"=[], "Override Limits?"=[]} ("Angular Accelerations"), "Angular \nAccelerations"=w406, "Override Limits?"=w405) -> (w404:T2)
            n161 = Read from Binary File(5:w415, 11:w414) -> (3:w413:refnum<file>)  [unwired: 4 in, 3 out]
          }
          frame "2.6" {
            n162 = Read from Binary File(5:w427, 11:w438) -> (2:w439:T17, 3:w437:refnum<file>)  [unwired: 4 in, 2 out]
            n163 = Unbundle(w439) -> ("Sample Period (s)"=w429:dbl, "Limits"=w428:T3, "Conditions"=w426:T4, "Angular Accelerations"=w425:T2)
            n164 = Read from Binary File(5:w436, 11:w437) -> (2:w435:cluster{"x":dbl, "y":dbl, "th":dbl}[], 3:w433:refnum<file>)  [unwired: 4 in, 2 out]
            n165 = Read from Binary File(5:w434, 11:w433) -> (2:w424:T7, 3:w431:refnum<file>)  [unwired: 4 in, 2 out]
            n166 = Read from Binary File(5:w432, 11:w431) -> (3:w430:refnum<file>)  [unwired: 4 in, 3 out]
          }
          frame "2.7" {
            n167 = Read from Binary File(5:w447, 11:w457) -> (2:w458:T17, 3:w456:refnum<file>)  [unwired: 4 in, 2 out]
            n168 = Unbundle(w458) -> ("Sample Period (s)"=w449:dbl, "Limits"=w448:T3, "Conditions"=w446:T4, "Angular Accelerations"=w445:T2)
            n169 = Read from Binary File(5:w455, 11:w456) -> (2:w454:cluster{"x":dbl, "y":dbl, "th":dbl}[], 3:w452:refnum<file>)  [unwired: 4 in, 2 out]
            n170 = Read from Binary File(5:w453, 11:w452) -> (2:w444:T7, 3:w450:refnum<file>)  [unwired: 4 in, 2 out]
            n171 = Read from Binary File(5:w451, 11:w450) -> (3:w443:refnum<file>)  [unwired: 4 in, 3 out]
            n172 = Read from Binary File(5:T15 [] ("Commands"), 11:w443) -> (2:w441:T15, 3:w442:refnum<file>)  [unwired: 4 in, 2 out]
          }
        }
        n173 = local write "Commands"(w326) -> ()
        n174 = Bundle("Sample Period (s)"=w333, "Limits"=w332, "Conditions"=w331, "Angular Accelerations"=w330) -> (w329:T17)  [unwired: 1 in]
        n175 = local write "Sample Period (s)"(w333) -> ()
        n176 = local write "Limits"(w332) -> ()
        n177 = local write "Conditions"(w331) -> ()
        n178 = local write "Angular Accelerations"(w330) -> ()
        n179 = Close File(refnum=w337) -> ()  [unwired: 1 in, 2 out]
        n180 = Bundle("Trajectory Data"=w327, "Points"=w325, w329) -> (w328:T24)  [unwired: 1 in]
      }
      event "Picture": Mouse Move; "Picture": Mouse Up {
        n181 = event-data() -> ("Type"=w472:T16, "Coords"=w475:T18)  [unwired: 1 in]
        n182 = Unbundle(w460) -> ("Drag Object"=w459:cluster{"Index":i32, "x":dbl, "y":dbl})  [unwired: 1 out]
        n183 = Unbundle(w465) -> ("Updated Waypoints"=w464:cluster{"x":dbl, "y":dbl, "th":dbl}[])  [unwired: 2 out]
        n184 = Unbundle(w459) -> ("Index"=w471:i32)  [unwired: 2 out]
        n185 = case shown="Default" w471 {
          selector: w471 -> [w485 _]
          tunnel: w475 -> [w494 w501]
          tunnel: w474 -> [w480 w500]
          tunnel: [w492 w499] -> w462
          tunnel: [w489 w498] -> w473
          tunnel: w464 -> [w490 w498]
          tunnel: [w486 w497] -> w463
          tunnel: w459 -> [w476 w497]
          tunnel: w472 -> [w487 _]
          tunnel: "Snap to foot" -> [w482 _]
          tunnel: "Snap robot to baseline" -> [w483 _]
          tunnel: "Angle Limiter" -> [w484 _]
          frame Default {
            # "Mouse up changes indes to break tracking,\notherwise update coords"
            n186 = property on="Picture" class="Pict"() -> ("Position"=w495:T20, "Draw Area Size"=w496:T21)  [unwired: 2 in, 2 out]
            n187 = Bundle("Snap robot to baseline"=w483, "Snap to foot"=w482, "Angle Limiter"=w484) -> (w481:T25)  [unwired: 1 in]
            n188 = call "Map to Feet.vi"("Draw Area Size"=w496, "Position"=w495, "Coords (px)"=w494) -> ("Point (ft)"=w493:cluster{dbl, dbl})  [unwired: 8 in]
            n189 = Equal?(x=lveventtype."Mouse Up" ("Type"), y=w487) -> (x = y?=w479:bool)
            n190 = call "Handle Pos and Rot.vi"("Mouse Up"=w479, "Picture in"=w480, "Option"=w481, "Coord (ft)"=w493, "Index"=w485, "Points in"=w490) -> ("Points out"=w489:cluster{"x":dbl, "y":dbl, "th":dbl}[])  [unwired: 5 in]
            n191 = Bundle(cluster=w476, "Index"=-1) -> (w477:cluster{"Index":i32, "x":dbl, "y":dbl})  [unwired: 2 in]
            n192 = Bundle(w485, "Pt Test Results"=enum16{"Miss", "Rect Hit", "Arrow Hit"}."Rect Hit") -> (w492:T26)  [unwired: 1 in]
            n193 = Select(t=w477, s=w479, f=w476) -> (s? t:f=w486:cluster{"Index":i32, "x":dbl, "y":dbl})
          }
          frame -1 {
            n194 = call "Point Test Shapes.vi"("Coords"=w501, "Points"=w498, "Picture in"=w500) -> ("Results"=w499:T8)  [unwired: 7 in, 1 out]
          }
        }
        n195 = Bundle("Drag Object"=w463, "Results"=w462) -> (w461:T27)  [unwired: 1 in]
      }
      event "Save": Value Change {
        n196 = event-data() -> ()  [unwired: 1 in, 1 out]
        n197 = Unbundle(w513) -> ("Updated Waypoints"=w510:cluster{"x":dbl, "y":dbl, "th":dbl}[], "Cluster"=w512:T17)  [unwired: 1 out]
        n198 = local read "folder names"() -> (w509:cluster{"name":string, "name":string})
        n199 = Unbundle(w509) -> ("name"=w504:string, "name"=w508:string)
        n200 = Empty String/Path?(string/path=w504) -> (empty?=w505:bool)
        n201 = case shown="False" w505 {
          tunnel: w504 -> [_ w530]
          tunnel: [w527 w529] -> w502
          tunnel: w503 -> [w527 w528]
          frame True {
          }
          frame False {
            n202 = Build Path(base path=w528, name or relative path=w530) -> (appended path=w529:path)
          }
        }
        n203 = Build Path(base path=w502, name or relative path=w508) -> (appended path=w507:path)
        n204 = Build Path(base path=w507, name or relative path="Filename") -> (appended path=w521:path)
        n205 = Write to Binary File(file (use dialog)=w521, data="2.7") -> (refnum out=w520:refnum<file>)  [unwired: 4 in, 2 out]
        n206 = Write to Binary File(file (use dialog)=w520, data=w512) -> (refnum out=w525:refnum<file>)  [unwired: 4 in, 2 out]
        n207 = Write to Binary File(file (use dialog)=w525, data=w510) -> (refnum out=w524:refnum<file>)  [unwired: 4 in, 2 out]
        n208 = Write to Binary File(file (use dialog)=w524, data=w517) -> (refnum out=w523:refnum<file>)  [unwired: 4 in, 2 out]
        n209 = Bundle("Trajectory Data"=w517, "Updated Waypoints"=w510, "Cluster"=w512) -> (w518:T28)  [unwired: 1 in]
        n210 = Write to Binary File(file (use dialog)=w523, data=w522) -> (refnum out=w516:refnum<file>)  [unwired: 4 in, 2 out]
        n211 = Write to Binary File(file (use dialog)=w516, data="Commands") -> (refnum out=w515:refnum<file>)  [unwired: 4 in, 2 out]
        n212 = Close File(refnum=w515) -> ()  [unwired: 1 in, 2 out]
      }
      event "Time (s)", "Snap to foot", "Angle Limiter", "Snap robot to baseline", "Limits", "Sample Period (s)", "Center Flip", "Conditions", "Commands", "Unjank", "Angular Accelerations": Value Change {
        # "Changes to any of these control will run the diagram to update the preview"
        n213 = event-data() -> ("CtlRef"=w541:refnum<vi>)  [unwired: 1 in]
        n214 = control-ref of="Center Flip"() -> (w542:refnum<vi>)
        n215 = Equal?(x=w542, y=w541) -> (x = y?=w540:bool)
        n216 = case shown="True" "Unjank" {
          tunnel: w535 -> [_ w547]
          tunnel: "Turn \nAcceleration" -> [_ w545]
          tunnel: "Turn \nDeceleration" -> [_ w544]
          frame False {
          }
          frame True {
            n217 = call "Turn Smother.vi"("Ignore Deceleration"=w544, "Ignore Acceleration"=w545, "input cluster"=w547) -> ("Angular Accelerations"=w546:T2)
            n218 = local write "Angular Accelerations"(w546) -> ()
          }
        }
        n219 = Unbundle(w535) -> ("Updated Waypoints"=w534:cluster{"x":dbl, "y":dbl, "th":dbl}[])  [unwired: 2 out]
        n220 = case shown="True" w540 {
          tunnel: w534 -> [w548 w550]
          tunnel: [w548 w549] -> w543
          frame False {
          }
          frame True {
            n221 = for {
              tunnel: w550 -> [w558] mode=indexing
              tunnel: [w551] -> w549 mode=indexing
              n222 = Unbundle(w558) -> ("x"=w557:dbl, "y"=w553:dbl, "th"=w552:dbl)
              n223 = Negate(x=w557) -> (-x=w556:dbl)
              n224 = Add(x=27.0 ("y"), y=w556) -> (x+y=w554:dbl)
              n225 = Bundle(w554, "y"=w553, "th"=w552) -> (w551:cluster{dbl, "y":dbl, "th":dbl})  [unwired: 1 in]
            }
          }
        }
      }
      event Key Down?; event type 5.0.x8000000b {
        n226 = event-data() -> ("VKey"=w569:T29)  [unwired: 1 in]
        n227 = local read "Snap robot to baseline"() -> (w576:bool)
        n228 = Unbundle(w563) -> ("Updated Waypoints"=w562:cluster{"x":dbl, "y":dbl, "th":dbl}[])  [unwired: 2 out]
        n229 = local read "Angle Limiter"() -> (w574:enum16{"90", "45", "15", "1"})
        n230 = local read "Snap to foot"() -> (w575:bool)
        n231 = Unbundle(w560) -> ("Hover Object"=w561:T8)  [unwired: 1 out]
        n232 = case shown="\"Down\"" w569 {
          tunnel: [cluster{dbl, dbl} {0.0, 0.0} ("Coord (ft)") cluster{dbl, dbl} {0.0, 0.1} ("Coord (ft)") cluster{dbl, dbl} {0.0, -0.1} ("Coord (ft)") cluster{dbl, dbl} {-0.1, 0.0} ("Coord (ft)") cluster{dbl, dbl} {0.1, 0.0} ("Coord (ft)")] -> w571
          tunnel: [_ w589 w591 w593 w595] -> w567
          tunnel: TRUE ("Delta") -> [_ w589 w591 w593 w595]
          frame Default {
          }
          frame "Up" {
          }
          frame "Down" {
          }
          frame "Left" {
          }
          frame "Right" {
          }
        }
        n233 = Unbundle(w561) -> ("Index"=w559:i32, "Pt Test Results"=w568:enum16{"Miss", "Rect Hit", "Arrow Hit"})
        n234 = Bundle("Snap robot to baseline"=w576, "Snap to foot"=w575, "Angle Limiter"=w574) -> (w573:T25)  [unwired: 1 in]
        n235 = case shown="\"Rect Hit\", Default" w568 {
          tunnel: [w579 w587] -> w577
          tunnel: w564 -> [_ w586]
          tunnel: w573 -> [_ w585]
          tunnel: w562 -> [w579 w584]
          tunnel: TRUE ("Delta") -> [_ w583]
          tunnel: w571 -> [_ w582]
          tunnel: w567 -> [_ w581]
          tunnel: [_ w581] -> w566
          tunnel: w559 -> [_ w580]
          frame "Miss" {
          }
          frame "Rect Hit", Default {
            n236 = call "Handle Pos and Rot.vi"("Delta"=w583, "Picture in"=w586, "Option"=w585, "Coord (ft)"=w582, "Index"=w580, "Points in"=w584) -> ("Points out"=w587:cluster{"x":dbl, "y":dbl, "th":dbl}[])  [unwired: 5 in]
          }
        }
        n237 = event-data("Discard?"=w566) -> ()  [unwired: 1 in, 1 out]
      }
      event "Play": Value Change {
        n238 = event-data() -> ()  [unwired: 1 in, 1 out]
        n239 = Unbundle(w599) -> ("Updated Waypoints"=w598:cluster{"x":dbl, "y":dbl, "th":dbl}[])  [unwired: 2 out]
        n240 = Tick Count (ms)() -> (millisecond timer value=w600:u32)
        n241 = Generate User Event(user event=w602, event data cluster=w600) -> ()  [unwired: 2 in, 2 out]
      }
      event User Event {
        n242 = event-data() -> ("Data"=w613:i32)  [unwired: 1 in]
        n243 = Unbundle(w606) -> ("Updated Waypoints"=w605:cluster{"x":dbl, "y":dbl, "th":dbl}[])  [unwired: 2 out]
        n244 = Tick Count (ms)() -> (millisecond timer value=w616:u32)
        n245 = Subtract(x=w616, y=w613) -> (x-y=w615:u32)
        n246 = Multiply(x=w615, y=0.001) -> (x*y=w612:dbl)
        n247 = local read "Duration (s)"() -> (w618:dbl)
        n248 = Quotient & Remainder(x=w612, y=0.02) -> (floor(x/y)=w610:dbl)  [unwired: 1 out]
        n249 = Multiply(x=0.02, y=w610) -> (x*y=w609:dbl)
        n250 = Less Or Equal?(x=w609, y=w618) -> (x <= y?=w619:bool)
        n251 = case shown="True" w619 {
          tunnel: w620 -> [_ w624]
          tunnel: w613 -> [_ w622]
          tunnel: w609 -> [_ w623]
          frame False {
          }
          frame True {
            n252 = local write "Time (s)"(w623) -> ()
            n253 = Generate User Event(user event=w624, event data cluster=w622) -> ()  [unwired: 2 in, 2 out]
          }
        }
        n254 = Wait (ms)(milliseconds to wait=u32 50) -> ()  [unwired: 1 out]
      }
      event "Directory": Value Change {
        n255 = event-data() -> ()  [unwired: 1 in, 1 out]
        n256 = Unbundle(w635) -> ("Updated Waypoints"=w634:cluster{"x":dbl, "y":dbl, "th":dbl}[])  [unwired: 2 out]
        n257 = call "File Dialog"("start path"=w627, "prompt"="Path Folder", "button label"="Select") -> ("selected path"=w626:path, "error out"=w628:errorcluster)  [unwired: 9 in, 2 out]
        n258 = Select(t=w627, s=w628, f=w626) -> (s? t:f=w625:path)
        n259 = Format Into String(format string=w631, w625) -> (resulting string=w632:string)  [unwired: 2 in, 1 out]
        n260 = property class="VI"("Front Panel.Title"=w632) -> ()  [unwired: 2 in, 2 out]
      }
    }
    n261 = feedback-in #1(w50) -> ()
    n262 = flat-sequence {
      tunnel: ["Time (s)"] -> w74
      tunnel: ["Sample Period (s)"] -> w27
      tunnel: ["Limits"] -> w56
      tunnel: ["Conditions"] -> w53
      tunnel: [w81] -> w28
      tunnel: ["Angular Accelerations"] -> w45
      tunnel: w44 -> [_]
      frame #0 {
        n263 = local read "Commands"() -> (w81:T5)
      }
    }
    n264 = control-ref of="Angular Accelerations"() -> (w43:refnum<vi>)
    n265 = call "Enforce Robot Rules.vi"("Clust Refnum"=w43, "Disable"=w65, "New Points"=w67, "Original Points"=w66) -> ("Points out"=w44:cluster{"x":dbl, "y":dbl, "th":dbl}[])  [unwired: 7 in]
    "WayPoints" <- w44
    n266 = Divide(x=w74, y=w27) -> (x/y=w63:dbl)
    n267 = Bundle("Sample Period (s)"=w27, "Limits"=w56, "Conditions"=w53, "Angular Accelerations"=w45) -> (w52:T17)  [unwired: 1 in]
    n268 = call "GenNewTraj.vi"("Parameters"=w52, "Points in"=w44) -> ("Time (s)"=w51:dbl, "Valid"=w29:bool, "Trajectory Data"=w42:T7, "Updated Waypoints"=w54:cluster{"x":dbl, "y":dbl, "th":dbl}[], "Distance (ft)"=w55:dbl)  [unwired: 5 in]
    "Duration (s)" <- w51
    "Distance (ft)" <- w55
    n269 = property on="Time (s)" class="Slide (strict)"("Scale.Maximum"=w51) -> ()  [unwired: 2 in, 2 out]
    n270 = Bundle("Time (s)"=w51, "Distance (ft)"=w55) -> (w69:cluster{"Time (s)":dbl, "Distance (ft)":dbl})  [unwired: 1 in]
    n271 = Bundle("Trajectory Data"=w42, "Updated Waypoints"=w54, w52) -> (w47:T30)  [unwired: 1 in]
    n272 = call "Draw Trajectory.vi"("Robot Index"=w63, "new picture in"=picture data[5B] ("new picture"), "Trajectory Data"=w42, "Picture in"=w77) -> ("Path Points"=w57:cluster{"x":dbl, "y":dbl}[], "Output Point"=w73:T31, "new picture"=w75:picture)  [unwired: 5 in]
    n273 = Unbundle(w40) -> ("Hover Object"=w39:T8)  [unwired: 1 out]
    n274 = call "Draw Shapes.vi"("Path Points"=w57, "Sample Period (s)"=w27, "Output Point"=w73, "Commands"=w28, "Results"=w39, "new picture in"=w75, "Points"=w54, "Picture in"=w77) -> ("new picture out"=→"Picture":picture)  [unwired: 3 in]
    n275 = call "Saved Checker.vi"("comp A"=w58, "comp B"=w47) -> ("Unsaved"=w33:bool)
    n276 = Select(t=0, s=w34, f=2000) -> (s? t:f=w35:i32)
    n277 = call "Update Annotations.vi"("Sample Period"=w27, "Commands"=w28, "Trajectory Data"=w42, "Robot Pt Index"=w63) -> ("Velocity Trace"=→"fps":dbl[], "Annotation Data"=w62:T32)  [unwired: 6 in]
    n278 = Select(t=cluster{u32, u32}[] [{14869218, 14869218}] ("Colors [4]"), s=w29, f=cluster{u32, u32}[] [{6094681, 6094681}] ("Colors [4]")) -> (s? t:f=w32:cluster{u32, u32}[])
    n279 = property on="Save" class="Bool"("Visible"=w33) -> ()  [unwired: 2 in, 2 out]
    n280 = property on="Unjank" class="Bool"("Colors [4]"=w32) -> ()  [unwired: 2 in, 2 out]
    n281 = property on="fps" class="WFGraph (strict)"("AnntList"=w62) -> ()  [unwired: 2 in, 2 out]
  }
  n282 = Format Into String(format string=w5, w1) -> (resulting string=w6:string)  [unwired: 2 in, 1 out]
  n283 = property class="VI"("Front Panel.Title"=w6) -> ()  [unwired: 2 in, 2 out]
